vi "Reshape acquired data.vi"(8 "error in (no error)":errorcluster, 9 "Array in":waveform(dbl)[](array[waveform]), 10 "data":waveform(dbl)[][](array[waveform]), 11 "Array 4":refnum<k21>[](array[refnum])) -> (0 "error out":errorcluster, 2 "Array out":waveform(dbl)[](array[waveform]), 3 "Array 3":refnum<k21>[](array[refnum]))   [LabVIEW 2016]
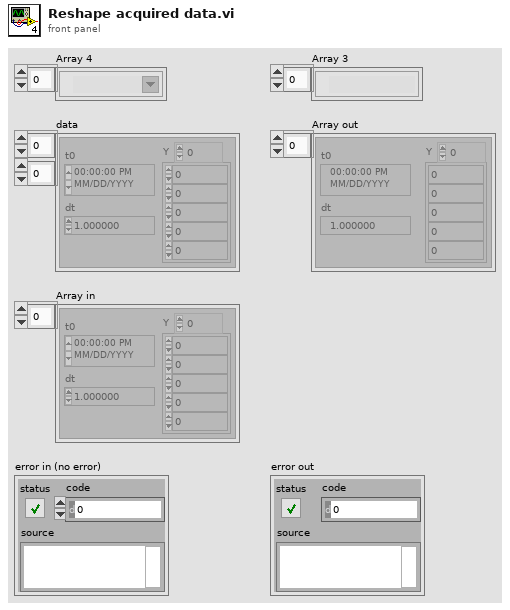
[diagram p1: front panel]
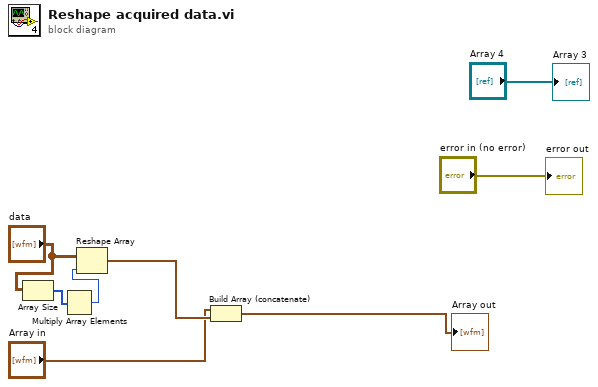
[diagram p0: block diagram]
diagram:
  n1 = Array Size(array="data") -> (size(s)=w5:i32[])
  n2 = Multiply Array Elements(1:w5) -> (0:w4:i32)
  n3 = Reshape Array("data", w4) -> (w3:waveform(dbl)[])
  n4 = Build Array (concatenate)("Array in", w3) -> (→"Array out":waveform(dbl)[])
  "Array 3" <- "Array 4"
  "error out" <- "error in (no error)"
